vi "Begin.vi"(8 "error in":errorcluster) -> (0 "error out":errorcluster)   [LabVIEW 2017]
doc: "Called before other user functions, this VI is expected to open initial I/O refnums, load in file data, and do all program initialization. Notice that the <B>error out</B> terminal is simply used for data flow. Wiring it to other structures or subVIs ensures that this VI runs first."
uses:
  <vilib>/Rock Robotics/SystemInterfaces/DIO/FPGA_DIOPWMChannel.ctl
  <vilib>/Rock Robotics/WPI/SafetyOutput/WPI_SafetyOutputConfigMenu.ctl
  <vilib>/Rock Robotics/WPI/DriverStation/WPI_DriverStationRobotMode2.ctl
  <vilib>/Rock Robotics/WPI/Joystick/WPI_JoystickDeviceEnum.ctl
  <vilib>/Rock Robotics/WPI/Solenoid/WPI_SolenoidChannel.ctl
  <vilib>/Rock Robotics/SystemInterfaces/DIO/FPGA_DIORelayChannel.ctl
  <vilib>/Rock Robotics/WPI/Relay/WPI_RelayDirection.ctl
  <vilib>/Rock Robotics/WPI/Relay/WPI_RelayValue.ctl
  Robot Global Data.vi
  <vilib>/Rock Robotics/Network Tables/NT Write String Array.vi
  <vilib>/Rock Robotics/WPI/Solenoid/WPI_SolenoidOpenDouble.vi
  <vilib>/Rock Robotics/WPI/MotorControl/WPI_MotorControlOpen VictorSP.vi
  <vilib>/Rock Robotics/WPI/MotorControl/WPI_MotorControlOpen SPARK.vi
  <vilib>/Rock Robotics/WPI/RobotDrive/WPI_RobotDriveOpen4MotorWithVictorSP.vi
  <vilib>/Rock Robotics/WPI/MotorControl/WPI_MotorControlOpen TalonSRX.vi
  <vilib>/Rock Robotics/WPI/Utilities/WPI_GetSetVariantRefNum.vi
  <vilib>/Rock Robotics/WPI/ThirdParty/Sensors/ADIS16448 IMU/ADIS16448_IMU.lvlib
panel:
  out "Sensor Ready?":bool
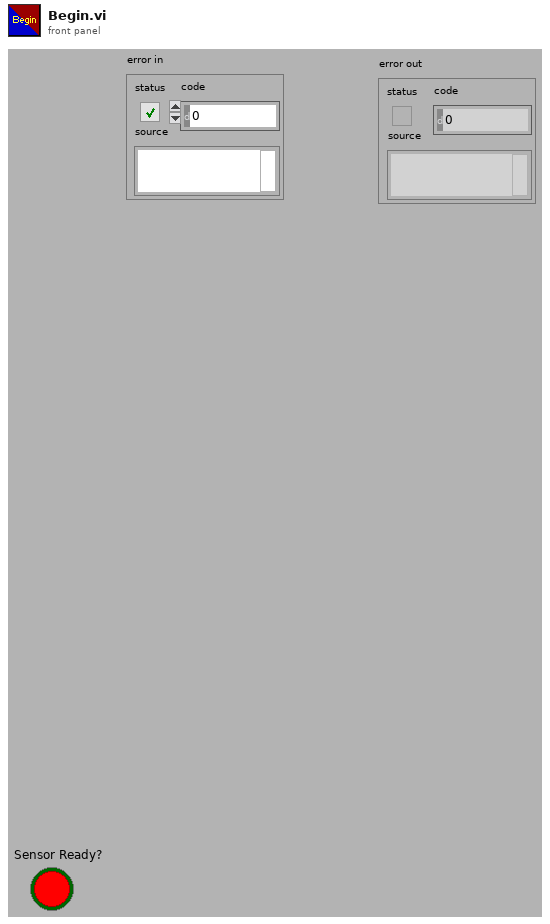
[diagram p1: front panel]
types:
  T1 = typedef "WPI_RelayValue.ctl" = enum16{"Off", "On", "Forward", "Reverse"}
  T2 = typedef "FPGA_DIOPWMChannel.ctl" = enum8{"PWM 0", "PWM 1", "PWM 2", "PWM 3", "PWM 4", "PWM 5", "PWM 6", "PWM 7", "PWM 8", "PWM 9", "PWM MXP 0", "PWM MXP 1", "PWM MXP 2", "PWM MXP 3", "PWM MXP 4", "PWM MXP 5", "PWM MXP 6", "PWM MXP 7", "PWM MXP 8", "PWM MXP 9", "Invalid"}
  T3 = typedef "WPI_RelayDirection.ctl" = enum16{"Both directions", "Forward only", "Reverse only"}
  T4 = typedef "FPGA_DIORelayChannel.ctl" = enum8{"Relay 0", "Relay 1", "Relay 2", "Relay 3", "Invalid"}
  T5 = typedef "WPI_JoystickDeviceEnum.ctl" = enum16{"USB 0", "USB 1", "USB 2", "USB 3", "USB 4", "USB 5"}
  T6 = typedef "WPI_SolenoidChannel.ctl" = enum8{"Solenoid 0", "Solenoid 1", "Solenoid 2", "Solenoid 3", "Solenoid 4", "Solenoid 5", "Solenoid 6", "Solenoid 7", "Invalid"}
  T7 = typedef "WPI_DriverStationRobotMode2.ctl" = enum16{"Autonomous Disabled", "Autonomous Enabled", "Teleop Disabled", "Teleop Enabled", "Disconnected", "Finish", "Test Disabled", "Test Enabled", "Emergency Stopped"}
  T8 = typedef "WPI_SafetyOutputConfigMenu.ctl" = enum16{"Enable", "Disable"}
  T9 = typedef "WPI_JoystickDevRef.ctl" = cluster{"Device":T5}
  T10 = typedef "WPI_MotorControlDeviceRef.ctl" = cluster{"DeviceStatus":errorcluster, "Type":T11, "PWM":cluster{"PWM Channel":T2, "DeadBand":T12}, "CAN":cluster{"Device Number":u8, "SetOutput VI Ref":variant, "GetOutput VI Ref":variant, "Enable VI Ref":variant, "Disable VI Ref":variant, "Data":variant}, "Invert":bool, "DIO PWM":cluster{"PWM \"Enable\" Channel":T2, "DIOChannel":T13, "PWM Rate":dbl}}
  T11 = typedef "WPI_MotorControlType.ctl" = enum16{"PWM", "CAN", "DIO PWM"}
  T12 = typedef "WPI_PWMDeadband.ctl" = cluster{"Name":string, "maxPositivePwm":i32, "minPositivePwm":i32, "centerPwm":i32, "maxNegativePwm":i32, "minNegativePwm":i32, "angularRange":u16}
  T13 = typedef "FPGA_DIOChannel.ctl" = enum8{"DIO 0", "DIO 1", "DIO 2", "DIO 3", "DIO 4", "DIO 5", "DIO 6", "DIO 7", "DIO 8", "DIO 9", "DIO MXP 0", "DIO MXP 1", "DIO MXP 2", "DIO MXP 3", "DIO MXP 4", "DIO MXP 5", "DIO MXP 6", "DIO MXP 7", "DIO MXP 8", "DIO MXP 9", "DIO MXP 10", "DIO MXP 11", "DIO MXP 12", "DIO MXP 13", "DIO MXP 14", "DIO MXP 15", "SPI Port CS1", "SPI Port CS2", "SPI Port CS3", "SPI Port MISO", "SPI Port MOSI", "Invalid"}
  T14 = typedef "WPI_RobotDriveDevRef.ctl" = cluster{"DevStatus":errorcluster, "Motors[]":T10[], "Square Inputs":bool, "Max Output":dbl}
  T15 = typedef "WPI_CompressorDevRef.ctl" = cluster{"DevStatus":errorcluster, "Pneumatics Control Module":u8}
  T16 = typedef "WPI_RelayDevRef.ctl" = cluster{"DevStatus":errorcluster, "Relay Channel":T4, "Relay Direction":T3}
  T17 = typedef "WPI_SolenoidDevRef.ctl" = cluster{"DevStatus":errorcluster, "Pneumatics Control Module":u8, "Forward Solenoid Channel":T6, "Reverse Solenoid Channel":T6}
  T18 = typedef "ADIS16448_IMU.lvlib/ADI_IMU_ADIS16448_IMUDevRef.ctl" = cluster{"DevStatus":errorcluster, "Handle":i32, "SPI Bus":T19, "Device Found":bool, "Device Ready":bool, "Yaw Axis":enum16{"X", "Y", "Z"}, "AHRS Algorithm":enum16{"Complementary", "Madgwick"}, "Serial":u16, "Lot ID 2":u16, "Lot ID 1":u16, "Bytes Per Sample":u16, "Calibrate On Open?":bool}
  T19 = typedef "spi_bus.ctl" = enum16{"SPI On-Board, CS0", "SPI On-Board, CS1", "SPI On-Board, CS2", "SPI On-Board, CS3", "SPI MXP", "Invalid"}
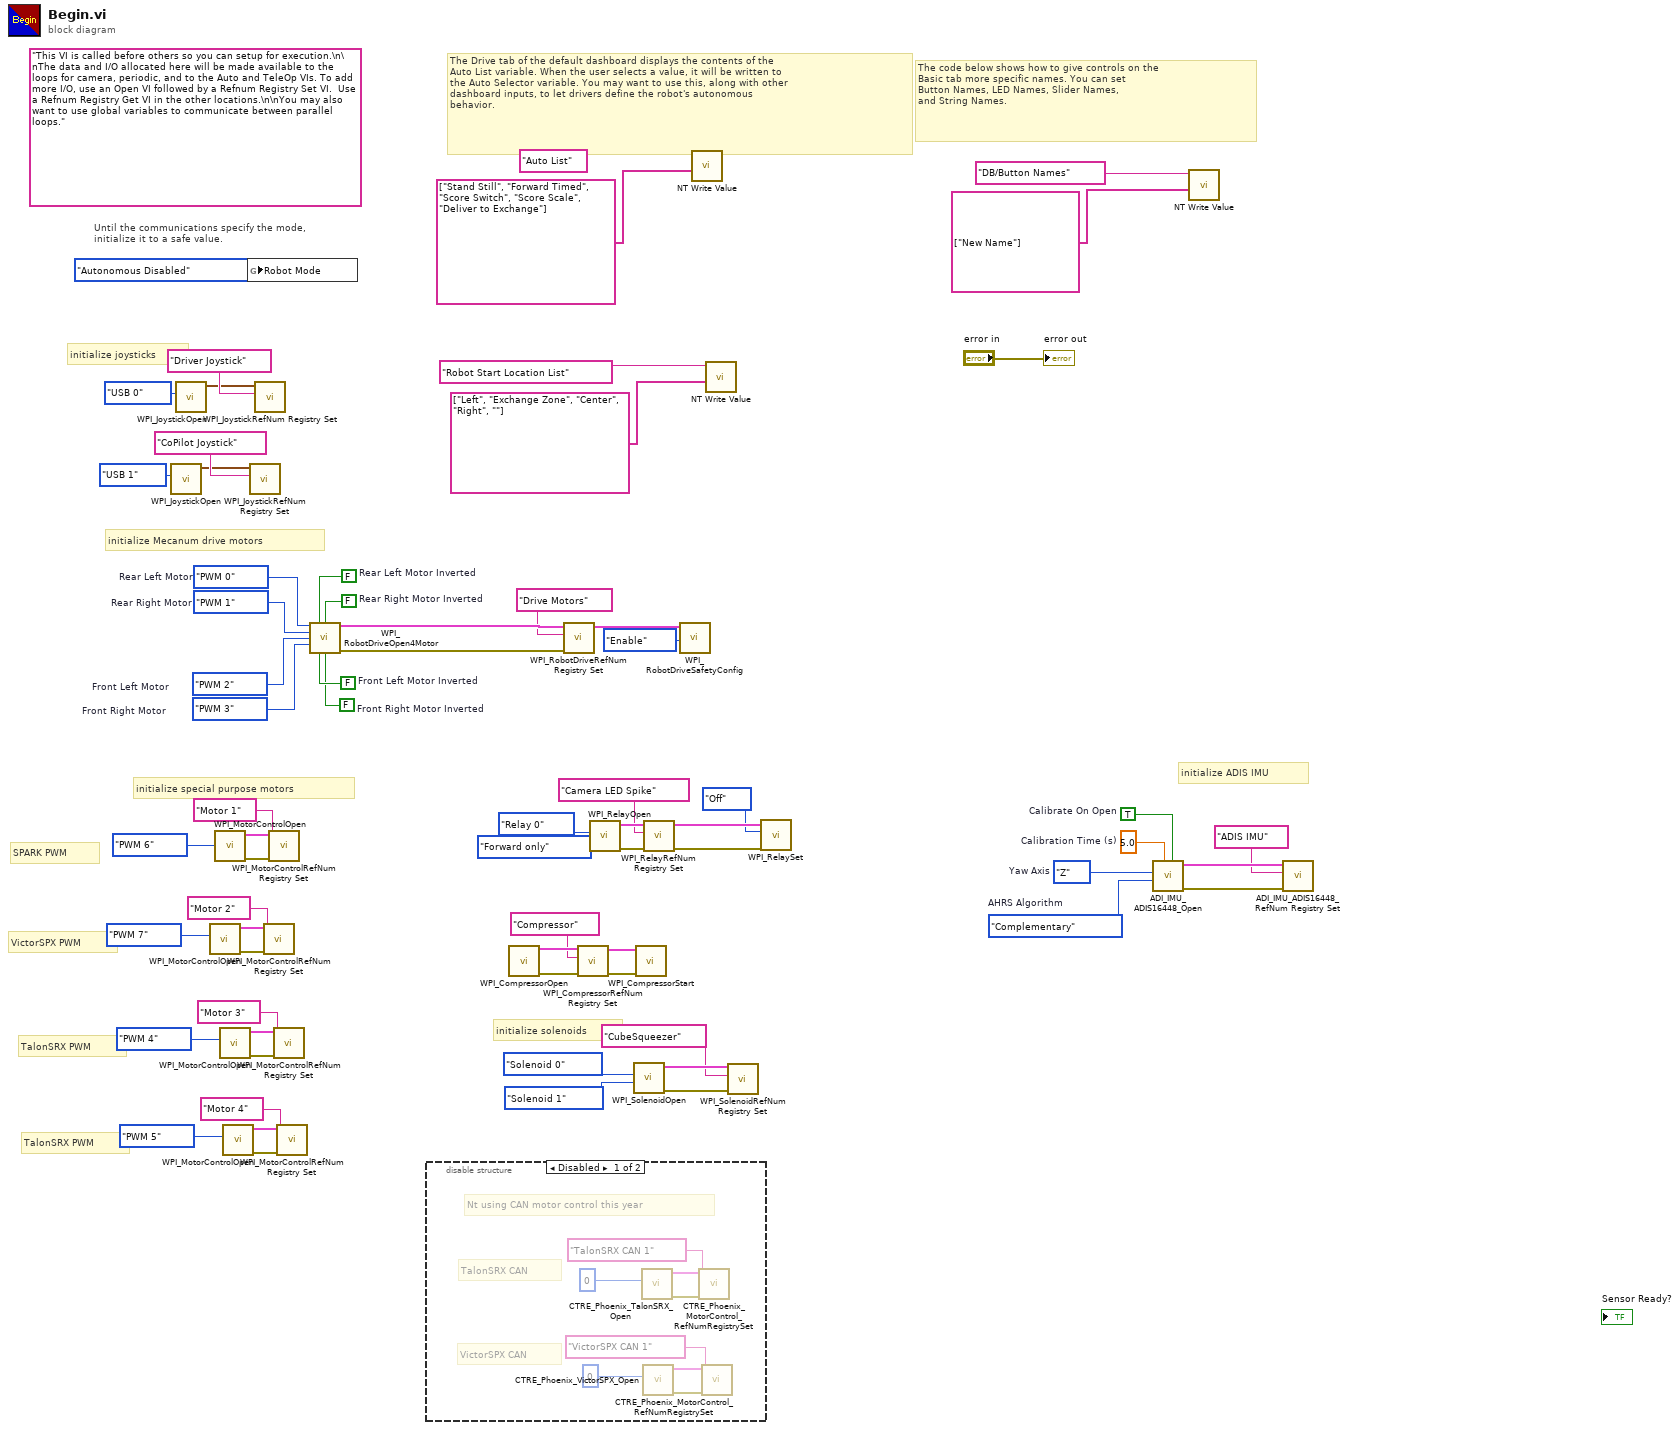
[diagram p0: block diagram]
diagram:
  w7 = TRUE  # Calibrate On Open
  w8 = 5.0  # Calibration Time (s)
  w9 = enum16{"Complementary", "Madgwick"}."Complementary"  # AHRS Algorithm
  w10 = enum16{"X", "Y", "Z"}."Z"  # Yaw Axis
  w32 = FALSE  # Rear Right Motor Inverted
  w33 = FALSE  # Rear Left Motor Inverted
  w34 = FALSE  # Front Right Motor Inverted
  w35 = FALSE  # Front Left Motor Inverted
  w51 = FPGA_DIOPWMChannel."PWM 3"  # Front Right Motor
  w52 = FPGA_DIOPWMChannel."PWM 2"  # Front Left Motor
  (unwired) "This VI is called before others so you can setup for execution.\n\nThe data and I/O allocated here will be made available to the loops for camera, periodic, and to the Auto and TeleOp VIs. To add more I/O, use an Open VI followed by a Refnum Registry Set VI.  Use a Refnum Registry Get VI in the other locations.\n\nYou may also want to use global variables to communicate between parallel loops."
  w64 = FPGA_DIOPWMChannel."PWM 1"  # Rear Right Motor
  w65 = FPGA_DIOPWMChannel."PWM 0"  # Rear Left Motor
  # "TalonSRX PWM"
  # "TalonSRX PWM"
  # "initialize ADIS IMU"
  # "SPARK PWM"
  # "VictorSPX PWM"
  # "initialize special purpose motors"
  # "initialize solenoids"
  # "The Drive tab of the default dashboard displays the contents of the\nAuto List variable. When the user selects a value, it will be written to\nthe Auto Selector variable. You may want to use this, along with other\ndashboard inputs, to let drivers define the robot's autonomous\nbehavior."
  # "The code below shows how to give controls on the\nBasic tab more specific names. You can set\nButton Names, LED Names, Slider Names,\nand String Names."
  # "initialize joysticks"
  # "Until the communications specify the mode,\ninitialize it to a safe value."
  # "initialize Mecanum drive motors"
  n1 = call <vilib>:"WPI_JoystickOpen.vi"("JoystickDevice"=WPI_JoystickDeviceEnum."USB 1") -> ("JoystickDevRef"=w30:T9)  [unwired: 10 in]
  n2 = call <vilib>:"WPI_JoystickOpen.vi"("JoystickDevice"=WPI_JoystickDeviceEnum."USB 0") -> ("JoystickDevRef"=w59:T9)  [unwired: 10 in]
  n3 = call-poly <vilib>:"WPI_MotorControlOpen.vi"("PWM Channel"=FPGA_DIOPWMChannel."PWM 7") -> ("error out"=w43:errorcluster, "MotorControlDeviceRef"=w42:T10)  [unwired: 9 in]
  n4 = call-poly <vilib>:"WPI_MotorControlOpen.vi"("PWM Channel"=FPGA_DIOPWMChannel."PWM 6") -> ("error out"=w41:errorcluster, "MotorControlDeviceRef"=w40:T10)  [unwired: 9 in]
  n5 = call-poly <vilib>:"WPI_MotorControlOpen.vi"("PWM Channel"=FPGA_DIOPWMChannel."PWM 4") -> ("error out"=w18:errorcluster, "MotorControlDeviceRef"=w17:T10)  [unwired: 9 in]
  n6 = call-poly <vilib>:"WPI_MotorControlOpen.vi"("PWM Channel"=FPGA_DIOPWMChannel."PWM 5") -> ("error out"=w14:errorcluster, "MotorControlDeviceRef"=w13:T10)  [unwired: 9 in]
  n7 = global write "Robot Global Data.vi" "Robot Mode"(WPI_DriverStationRobotMode2."Autonomous Disabled" ("Robot Mode")) -> ()
  n8 = call <vilib>:"WPI_JoystickRefNum Registry Set.vi"("refnum name"="CoPilot Joystick", "JoystickDevRef"=w30) -> ()  [unwired: 8 in, 2 out]
  n9 = call <vilib>:"WPI_JoystickRefNum Registry Set.vi"("refnum name"="Driver Joystick", "JoystickDevRef"=w59) -> ()  [unwired: 8 in, 2 out]
  n10 = call <vilib>:"WPI_MotorControlRefNum Registry Set.vi"("error in (no error)"=w43, "refnum name"="Motor 2", "MotorControlDevRef"=w42) -> ()  [unwired: 7 in, 2 out]
  n11 = call <vilib>:"WPI_MotorControlRefNum Registry Set.vi"("error in (no error)"=w41, "refnum name"="Motor 1", "MotorControlDevRef"=w40) -> ()  [unwired: 7 in, 2 out]
  n12 = call <vilib>:"WPI_MotorControlRefNum Registry Set.vi"("error in (no error)"=w18, "refnum name"="Motor 3", "MotorControlDevRef"=w17) -> ()  [unwired: 7 in, 2 out]
  n13 = call <vilib>:"WPI_MotorControlRefNum Registry Set.vi"("error in (no error)"=w14, "refnum name"="Motor 4", "MotorControlDevRef"=w13) -> ()  [unwired: 7 in, 2 out]
  n14 = call-poly <vilib>:"WPI_RobotDriveOpen4Motor.vi"("Rear Left Motor"=w65, "Rear Left Motor Inverted"=w33, "Rear Right Motor Inverted"=w32, "Rear Right Motor"=w64, "Front Left Motor"=w52, "Front Right Motor"=w51, "Front Left Motor Inverted"=w35, "Front Right Motor Inverted"=w34) -> ("RobotDriveDevRef"=w68:T14, "error out"=w66:errorcluster)  [unwired: 6 in]
  n15 = disable-structure shown="Disabled" {
    frame Disabled {
      # "Nt using CAN motor control this year"
      # "VictorSPX CAN"
      # "TalonSRX CAN"
      n16 = call <vilib>:"CTRE_Phoenix_TalonSRX_Open.vi"("Device Number"=u8 0) -> ("error out"=w74:errorcluster, "CAN Talon SRX Ref"=w73:T10)  [unwired: 9 in]
      n17 = call <vilib>:"CTRE_Phoenix_VictorSPX_Open.vi"("Device Number"=u8 0) -> ("error out"=w76:errorcluster, "CAN Talon SRX Ref"=w75:T10)  [unwired: 9 in]
      n18 = call <vilib>:"CTRE_Phoenix_MotorControl_RefNumRegistrySet.vi"("error in (no error)"=w74, "refnum name"="TalonSRX CAN 1", "PhoenixMotorControlDevRef"=w73) -> ()  [unwired: 7 in, 2 out]
      n19 = call <vilib>:"CTRE_Phoenix_MotorControl_RefNumRegistrySet.vi"("error in (no error)"=w76, "refnum name"="VictorSPX CAN 1", "PhoenixMotorControlDevRef"=w75) -> ()  [unwired: 7 in, 2 out]
    }
    frame Enabled {
    }
  }
  n20 = call <vilib>:"WPI_CompressorOpen.vi"() -> ("CompressorDevRef"=w25:T15, "error out"=w26:errorcluster)  [unwired: 14 in]
  n21 = call <vilib>:"WPI_RobotDriveRefNum Registry Set.vi"("error in (no error)"=w66, "refnum name"="Drive Motors", "RobotDriveDevRef"=w68) -> ("RobotDriveDevRef"=w63:T14)  [unwired: 1 in, 7 out]
  n22 = call <vilib>:"WPI_CompressorRefNum Registry Set.vi"("error in (no error)"=w26, "refnum name"="Compressor", "CompressorDevRef"=w25) -> ("error out"=w24:errorcluster, "CompressorDevRef"=w23:T15)  [unwired: 7 in]
  n23 = call <vilib>:"WPI_RelayOpen.vi"("Relay Direction"=WPI_RelayDirection."Forward only", "Relay Channel"=FPGA_DIORelayChannel."Relay 0") -> ("error out"=w28:errorcluster, "RelayDevRef"=w27:T16)  [unwired: 8 in]
  n24 = call-poly <vilib>:"WPI_SolenoidOpen.vi"("Reverse Solenoid Channel"=WPI_SolenoidChannel."Solenoid 1" ("Extend Solenoid Channel"), "Forward Solenoid Channel"=WPI_SolenoidChannel."Solenoid 0" ("Retract Solenoid Channel")) -> ("error out"=w46:errorcluster, "SolenoidDevRef"=w45:T17)  [unwired: 2 in, 6 out]
  n25 = call <vilib>:"WPI_CompressorStart.vi"("error in (no error)"=w24, "CompressorDevRef"=w23) -> ()  [unwired: 8 in, 2 out]
  n26 = call <vilib>:"WPI_RelayRefNum Registry Set.vi"("error in (no error)"=w28, "refnum name"="Camera LED Spike", "RelayDevRef"=w27) -> ("error out"=w3:errorcluster, "RelayDevRef"=w2:T16)  [unwired: 7 in]
  n27 = call <vilib>:"WPI_RobotDriveSafetyConfig.vi"("mode"=WPI_SafetyOutputConfigMenu."Enable", "RobotDriveDevRef"=w63) -> ()  [unwired: 8 in, 2 out]
  n28 = call-poly <vilib>:"NT Write Value.vi"("String Array"=string[] ["Stand Still", "Forward Timed", "Score Switch", "Score Scale", "Deliver to Exchange"], "Name"="Auto List") -> ()  [unwired: 9 in, 1 out]
  n29 = call-poly <vilib>:"NT Write Value.vi"("String Array"=string[] ["Left", "Exchange Zone", "Center", "Right", ""], "Name"="Robot Start Location List") -> ()  [unwired: 9 in, 1 out]
  n30 = call <vilib>:"WPI_SolenoidRefNum Registry Set.vi"("error in (no error)"=w46, "refnum name"="CubeSqueezer", "SolenoidDevRef"=w45) -> ()  [unwired: 7 in, 2 out]
  n31 = call <vilib>:"WPI_RelaySet.vi"("error in (no error)"=w3, "RelayValue"=WPI_RelayValue."Off", "RelayDevRef"=w2) -> ()  [unwired: 7 in, 2 out]
  n32 = call <vilib>:"ADI_IMU_ADIS16448_Open.vi"("Calibrate On Open"=w7, "Calibration Time (s)"=w8, "AHRS Algorithm"=w9, "Yaw Axis"=w10) -> ("error out"=w6:errorcluster, "ADI IMU DevRef Out"=w5:T18)  [unwired: 5 in, 1 out]
  n33 = call-poly <vilib>:"NT Write Value.vi"("String Array"=string[] ["New Name"], "Name"="DB/Button Names") -> ()  [unwired: 9 in, 1 out]
  n34 = call <vilib>:"ADI_IMU_ADIS16448_RefNum Registry Set.vi"("error in (no error)"=w6, "refnum name"="ADIS IMU", "ADI IMU DevRef"=w5) -> ()  [unwired: 7 in, 2 out]
  "error out" <- "error in"
